vi "Read Timed Out.vi"(8 "error in (no error)":errorcluster, 11 "Wait On Integer Step in":refnum<class "Wait On Integer Step.lvclass">) -> (0 "error out":errorcluster, 2 "Timed Out?":bool, 3 "Wait On Integer Step out":refnum<class "Wait On Integer Step.lvclass">)   [LabVIEW 2015, in "Wait On Integer Step.lvclass"]
uses:
  Wait On Integer Step.lvclass
  Wait On Integer Step.lvclass/Wait On Integer Step.ctl
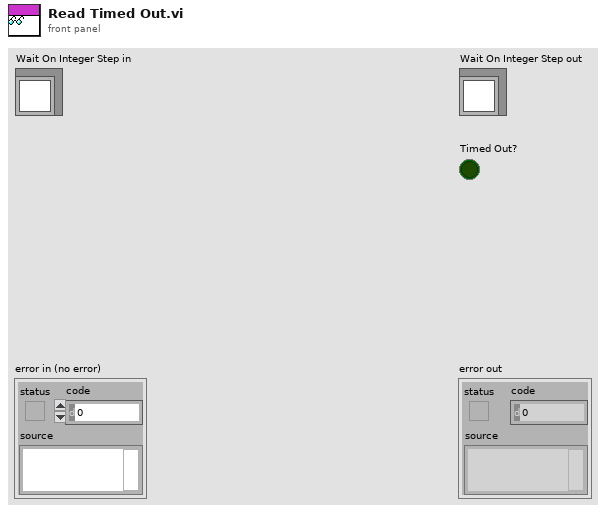
[diagram p1: front panel]
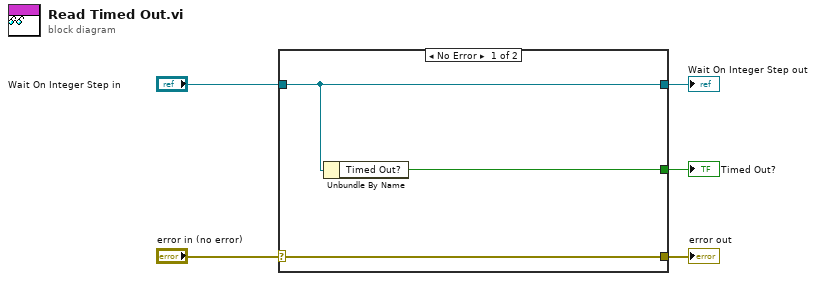
[diagram p0: block diagram]
diagram:
  n1 = case shown="No Error" "error in (no error)" {
    selector: "error in (no error)" -> [w8 w9]
    tunnel: [w8 w9] -> w4
    tunnel: [w7 w10] -> w2
    tunnel: "Wait On Integer Step in" -> [w7 w10]
    tunnel: [w6 _] -> w1
    frame No Error {
      n2 = Unbundle By Name(w7) -> ("Timed Out?"=w6:bool)
    }
    frame Error {
    }
  }
  "error out" <- w4
  "Wait On Integer Step out" <- w2
  "Timed Out?" <- w1
